vi "Proceed failed Msg.vi"(8 "error in (no error)":errorcluster, 10 "Return Msg":refnum<class "Return undeliverable Msg.lvclass">, 11 "Alice in":refnum<class "Alice.lvclass">) -> (0 "error out":errorcluster, 3 "Alice out":refnum<class "Alice.lvclass">)   [LabVIEW 2014, in "Alice.lvlib" / "Alice.lvclass"]
uses:
  Alice.lvclass
  Proxy/Proxy Messages/Return undeliverable Msg/Return undeliverable Msg.lvclass
  <vilib>/ActorFramework/Message Enqueuer/Message Priority.ctl
  <vilib>/ActorFramework/Message Enqueuer/Message Enqueuer.lvclass
panel:
  out "class name":string
  out "Message Priority":T1=enum."Normal"
  out "Tx Error":errorcluster
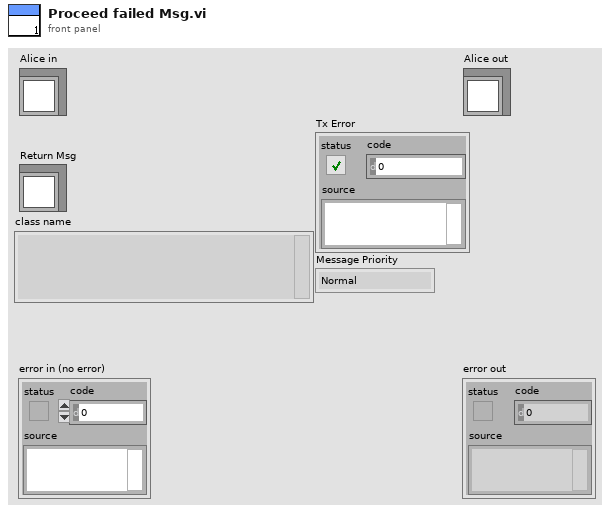
[diagram p1: front panel]
types:
  T1 = typedef "Actor Framework.lvlib/Message Enqueuer.lvclass/Message Priority.ctl" = enum16{"Low", "Normal", "High"}
  T2 = cluster{"Tx Message":refnum<class "Message.lvclass">, "Tx Error":errorcluster, "Message Priority":T1}
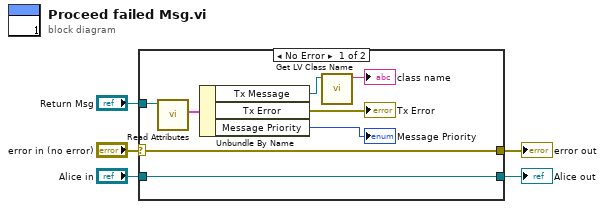
[diagram p0: block diagram]
diagram:
  n1 = case shown="No Error" "error in (no error)" {
    selector: "error in (no error)" -> [w12 w15]
    tunnel: [w12 w15] -> w4
    tunnel: [w13 w14] -> w2
    tunnel: "Alice in" -> [w13 w14]
    tunnel: "Return Msg" -> [w11 _]
    frame No Error {
      n2 = call "Read Attributes.vi"("Abstract Message Template in"=w11) -> ("Payload"=w10:T2)  [unwired: 9 in, 1 out]
      n3 = Unbundle By Name(w10) -> ("Tx Message"=w7:refnum<class "Message.lvclass">, "Tx Error"=→"Tx Error":errorcluster, "Message Priority"=→"Message Priority":T1)
      n4 = call <vilib>:"Get LV Class Name.vi"("object"=w7) -> ("class name"=→"class name":string)  [unwired: 9 in, 1 out]
    }
    frame Error {
    }
  }
  "error out" <- w4
  "Alice out" <- w2
